vi "Decode Data.vi"(8 "Error In":errorcluster, 10 "Response String":string, 11 "Open Weather Session In":refnum<class "Open Weather Session.lvclass">) -> (0 "Error Out":errorcluster, 2 "Raw Weather Data":T1, 3 "Open Weather Session Out":refnum<class "Open Weather Session.lvclass">)   [LabVIEW 2019, in "Open Weather Session.lvclass"]
uses:
  Open Weather Session.lvclass
  Controls/Raw Weather Data.ctl
  Controls/Weather Sample Raw Data.ctl
  Controls/Weather Description Raw Data.ctl
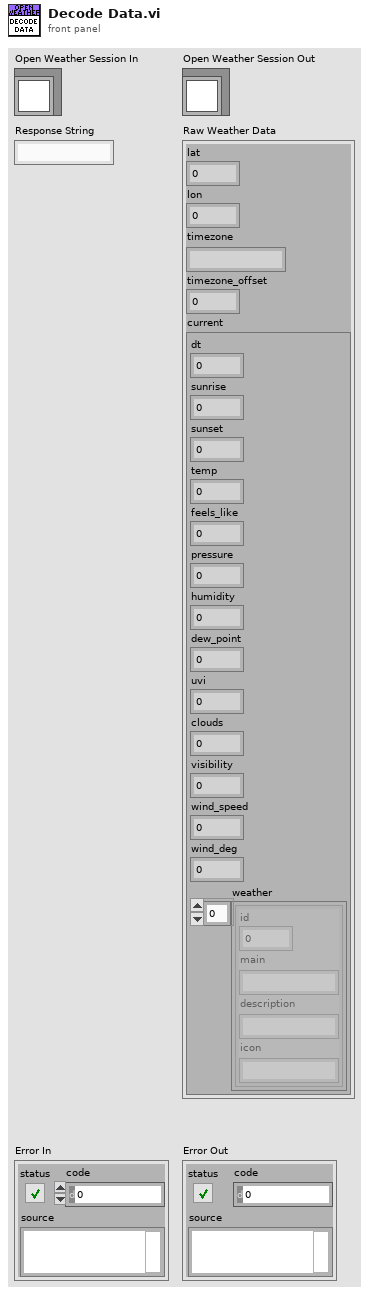
[diagram p1: front panel]
types:
  T1 = typedef "Open Weather Session.lvclass/Raw Weather Data.ctl" = cluster{"lat":dbl, "lon":dbl, "timezone":string, "timezone_offset":i32, "current":T2}
  T2 = typedef "Open Weather Session.lvclass/Weather Sample Raw Data.ctl" = cluster{"dt":i32, "sunrise":i32, "sunset":i32, "temp":dbl, "feels_like":dbl, "pressure":i32, "humidity":i32, "dew_point":dbl, "uvi":dbl, "clouds":i32, "visibility":i32, "wind_speed":dbl, "wind_deg":i32, "weather":T3[]}
  T3 = typedef "Open Weather Session.lvclass/Weather Description Raw Data.ctl" = cluster{"id":u32, "main":string, "description":string, "icon":string}
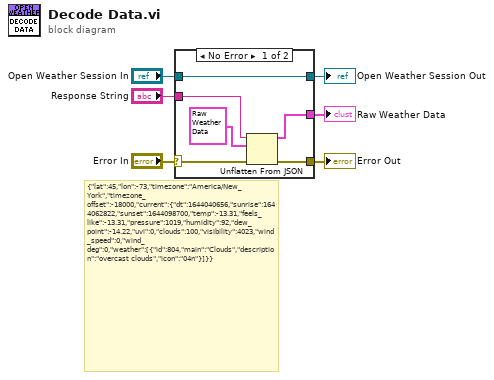
[diagram p0: block diagram]
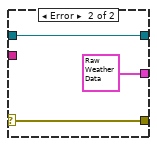
[diagram p2: hidden frame]
diagram:
  # "{\"lat\":45,\"lon\":-73,\"timezone\":\"America/New_York\",\"timezone_offset\":-18000,\"current\":{\"dt\":1644040656,\"sunrise\":1644062822,\"sunset\":1644098700,\"temp\":-13.31,\"feels_like\":-13.31,\"pressure\":1019,\"humidity\":92,\"dew_point\":-14.22,\"uvi\":0,\"clouds\":100,\"visibility\":4023,\"wind_speed\":0,\"wind_deg\":0,\"weather\":[{\"id\":804,\"main\":\"Clouds\",\"description\":\"overcast clouds\",\"icon\":\"04n\"}]}}"
  n1 = case shown="No Error" "Error In" {
    selector: "Error In" -> [w9 w14]
    tunnel: [w12 w15] -> w6
    tunnel: [w8 w14] -> w5
    tunnel: "Open Weather Session In" -> [w12 w15]
    tunnel: "Response String" -> [w11 _]
    tunnel: [w7 T1 {"lat"=0.0, "lon"=0.0, "timezone"="", "timezone_offset"=0, "current"={"dt"=0, "sunrise"=0, "sunset"=0, "temp"=0.0, "feels_like"=0.0, "pressure"=0, "humidity"=0, "dew_point"=0.0, "uvi"=0.0, "clouds"=0, "visibility"=0, "wind_speed"=0.0, "wind_deg"=0, "weather"=[]}} ("Raw Weather Data")] -> w1
    frame No Error {
      n2 = Unflatten From JSON(JSON string=w11, type and defaults=T1 {"lat"=0.0, "lon"=0.0, "timezone"="", "timezone_offset"=0, "current"={"dt"=0, "sunrise"=0, "sunset"=0, "temp"=0.0, "feels_like"=0.0, "pressure"=0, "humidity"=0, "dew_point"=0.0, "uvi"=0.0, "clouds"=0, "visibility"=0, "wind_speed"=0.0, "wind_deg"=0, "weather"=[]}} ("Raw Weather Data"), error in (no error)=w9) -> (value=w7:T1, error out=w8:errorcluster)  [unwired: 4 in]
    }
    frame Error {
    }
  }
  "Open Weather Session Out" <- w6
  "Error Out" <- w5
  "Raw Weather Data" <- w1
